vi "Main.vi"(11 "Module Admin":refnum<class "Delacor_lib_QMH_Cloneable Module Admin.lvclass">) -> ()   [LabVIEW 2020, in "FGen.lvlib"]
doc: "This template is based off of the Queued Message Handler design pattern and the Queued Message Handler project template that ships with LabVIEW.\n\nThe main difference is that the queue is private to this module and communication between modules is performed via Broadcast and Request events.\n\nRequest events are wrapped in public API methods and are handled in the Event Handling Loop (EHL) of this VI. Any module can register for Broadcast events sent by this module. The EHL generates messages based on user interface actions.\n\nThe Message Handling Loop (MHL) processes messages generated by the EHL, or by other messages. The messages are string values, so new messages can be added easily to the Message Cases case structure in the MHL. Each message cluster can also provide an optional value for Message Data, which is a variant that can be converted to whatever message-specific data is required.\n_____\nBased on DQMH Project Template 6.0.0.91."
uses:
  FGen.lvlib
  <vilib>/Delacor/Delacor QMH/Libraries/Message Queue_class/Delacor_lib_QMH_Message Queue.lvclass
  Module Data--cluster.ctl
  <vilib>/Utility/miscctls.llb/LVPointTypeDef.ctl
  <vilib>/Utility/error.llb/Error Cluster From Error Code.vi
  <vilib>/ErrorRing/Error Ring.xnode
  <vilib>/Delacor/Delacor QMH/Libraries/Message Queue_class/Delacor_lib_QMH_Enqueue Message (Single).vi
  Stop Argument--cluster.ctl
  <vilib>/Delacor/Delacor QMH/Libraries/Cloneable Module Admin_class/Delacor_lib_QMH_Cloneable Module Admin.lvclass
  Set Signal Type Argument--cluster.ctl
  Generador/Generador.lvclass
  Set to Default Argument--cluster.ctl
  Generate Signal (Reply Payload)--cluster.ctl
  Generate Signal Argument--cluster.ctl
panel:
  out "error out":errorcluster
  out "Status":string
  in  "Simulate EHL Error":bool
  in  "Simulate MHL Error":bool
  # "Other QMH Modules communicate with this Module via its Public API (wrappers for its Request Events).\n\nThis Module communicates with other Modules via its Broadcast Events.\nAny module that wants to get these messages, just registers for this module's Broadcast events."
  # "This template is for the Delacor Modified Queued Message Handler design pattern.\n\nSee the block diagram for more information on how to use this template."
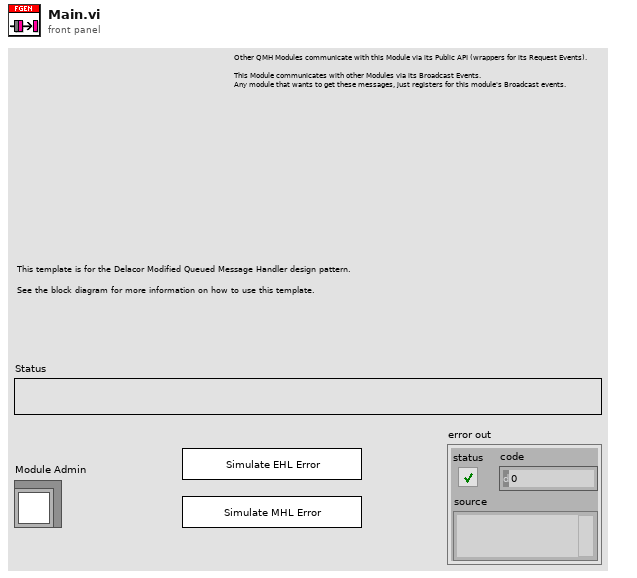
[diagram p1: front panel]
types:
  T1 = typedef "FGen.lvlib/Request Events--cluster.ctl" = cluster{"Stop Module":refnum<user-event>, "Show Panel":refnum<user-event>, "Hide Panel":refnum<user-event>, "Show Diagram":refnum<user-event>, "Get Module Execution Status":refnum<user-event>, "Set Signal Type":refnum<user-event>, "Set to Default":refnum<user-event>, "Generate Signal":refnum<user-event>}
  T2 = typedef "FGen.lvlib/Module Data--cluster.ctl" = cluster{"Status":string, "Generator":refnum<class "Generador.lvclass">}
  T3 = enum32{"invalid lock state", "Not Locked", "Locked (No Password)", "Password-protected"}
  T4 = typedef "FGen.lvlib/Stop Argument--cluster.ctl" = cluster{"Module ID":i32, "Origin":string, "Exit via Stop Module Req?":bool, "Wait for Module to stop?":bool}
  T5 = typedef "FGen.lvlib/Set Signal Type Argument--cluster.ctl" = cluster{"Module ID":i32, "signal type":enum16{"Sine Wave", "Triangle Wave", "Square Wave", "Sawtooth Wave"}}
  T6 = typedef "FGen.lvlib/Set to Default Argument--cluster.ctl" = cluster{"Module ID":i32, "Boolean":bool}
  T7 = typedef "FGen.lvlib/Generate Signal Argument--cluster.ctl" = cluster{"Module ID":i32, "Wait Notifier":refnum<notifier>, "wait for reply":bool}
  T8 = typedef "LVPointTypeDef.ctl" = cluster{"Horizontal":i16, "Vertical":i16}
  T9 = enum32{"Invalid", "Standard", "Closed", "Hidden", "Minimized", "Maximized"}
  T10 = typedef "FGen.lvlib/Generate Signal (Reply Payload)--cluster.ctl" = cluster{"signal out":waveform(dbl), "Generate Signal_error":errorcluster}
  T11 = enum16{"Sine Wave", "Triangle Wave", "Square Wave", "Sawtooth Wave"}
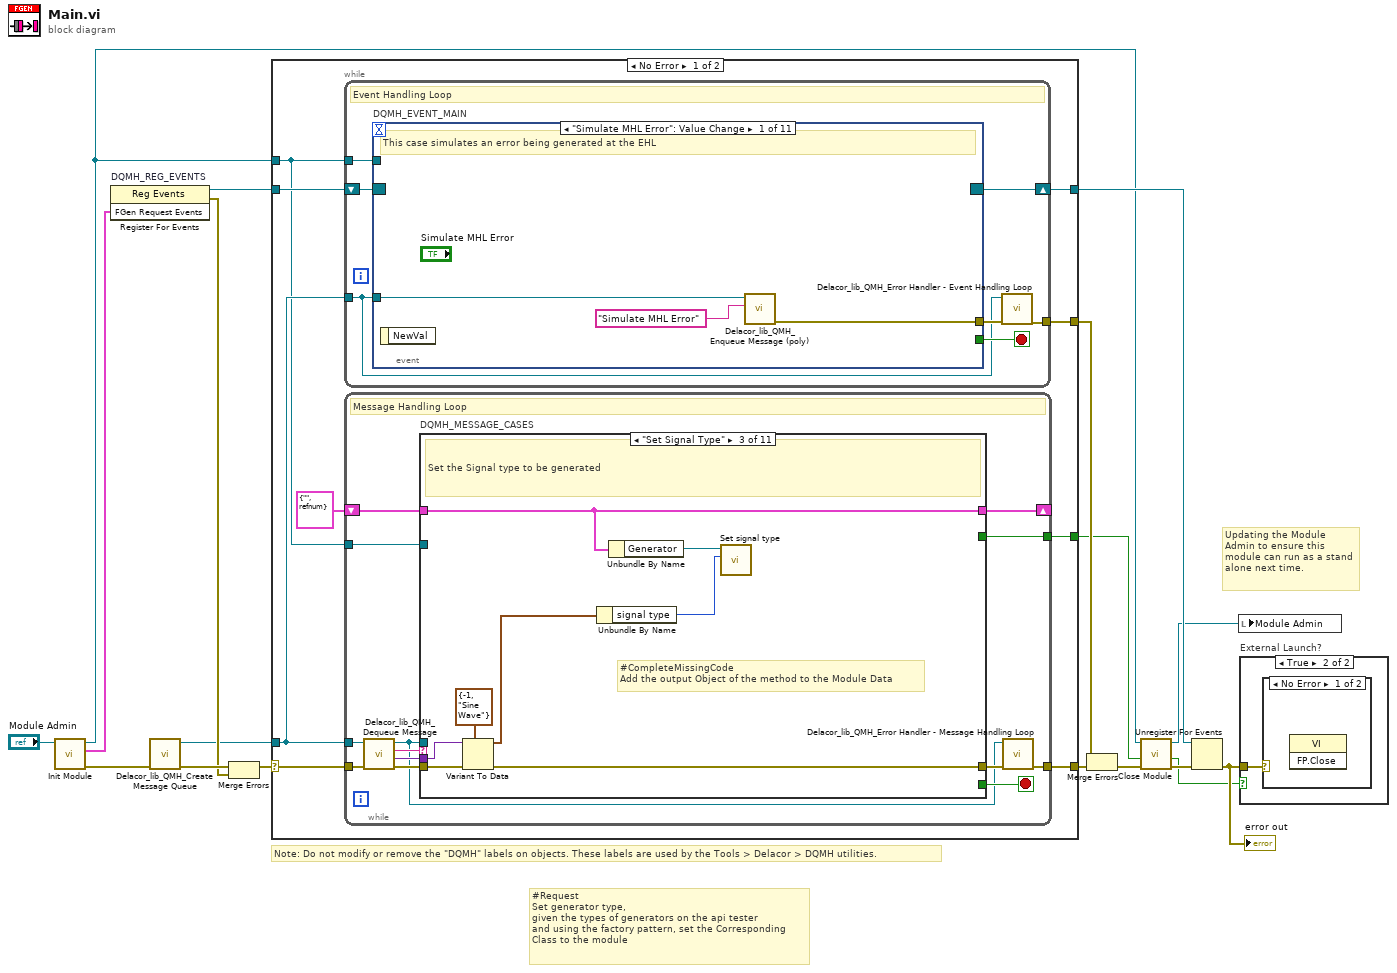
[diagram p0: block diagram]
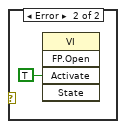
[diagram p3: hidden frame]
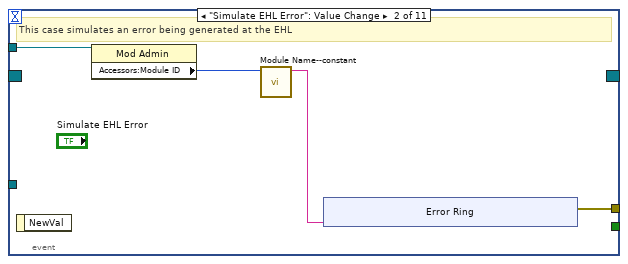
[diagram p4: hidden frame]
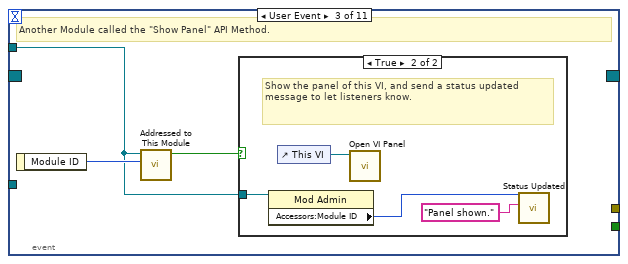
[diagram p5: hidden frame]
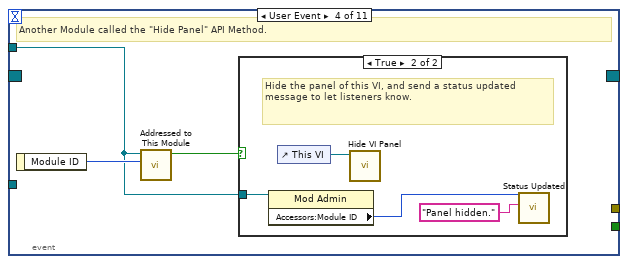
[diagram p7: hidden frame]
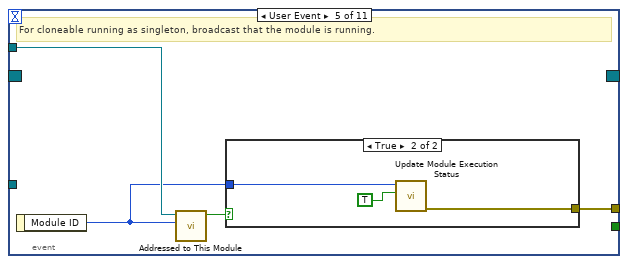
[diagram p9: hidden frame]
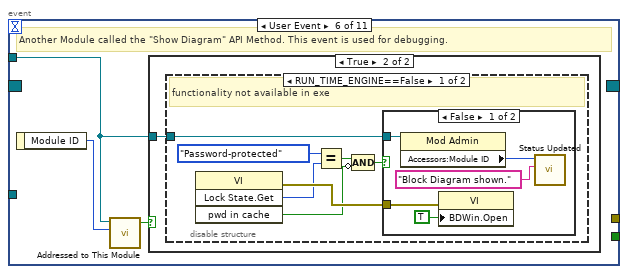
[diagram p11: hidden frame]
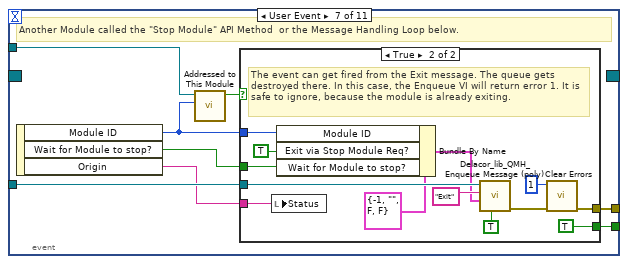
[diagram p15: hidden frame]
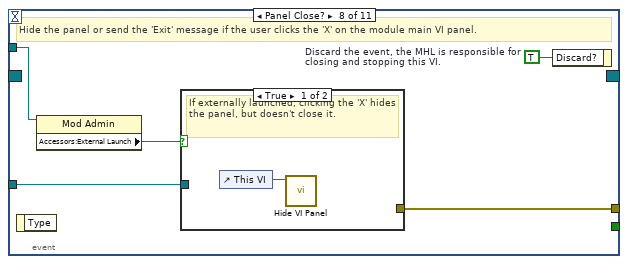
[diagram p17: hidden frame]
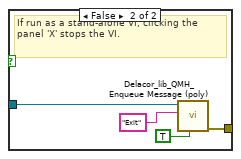
[diagram p18: hidden frame]
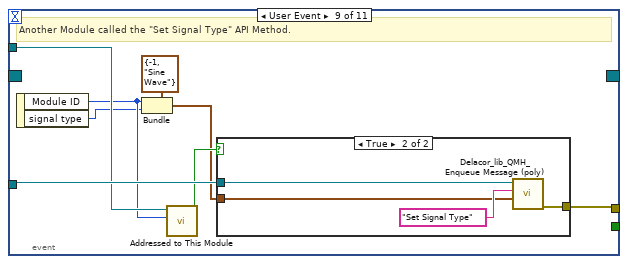
[diagram p19: hidden frame]
diagram:
  # "#Request\nSet generator type, \ngiven the types of generators on the api tester\nand using the factory pattern, set the Corresponding\nClass to the module"
  # "Note: Do not modify or remove the \"DQMH\" labels on objects. These labels are used by the Tools > Delacor > DQMH utilities."
  # "Updating the Module Admin to ensure this module can run as a stand alone next time."
  n1 = call "Init Module.vi"("Cloneable Module Admin in"="Module Admin") -> ("error out"=w15:errorcluster, "FGen Request Events"=w7:T1, "Cloneable Module Admin out"=w4:refnum<class "Delacor_lib_QMH_Cloneable Module Admin.lvclass">)  [unwired: 8 in]
  n2 = register-events "DQMH_REG_EVENTS"(w7) -> (reference out=w8:refnum<event-registration>, error out=w10:errorcluster)  [unwired: 2 in]
  n3 = call <vilib>:"Delacor_lib_QMH_Create Message Queue.vi"("error in"=w15) -> ("error out"=w12:errorcluster, "Message Queue"=w6:refnum<class "Delacor_lib_QMH_Message Queue.lvclass">)  [unwired: 9 in]
  n4 = Merge Errors(w12, w10) -> (w11:errorcluster)
  n5 = case shown="No Error" w11 {
    selector: w11 -> [w25 w290]
    tunnel: [w27 w289] -> w16
    tunnel: [w24 w297] -> w9
    tunnel: w8 -> [w22 w297]
    tunnel: w6 -> [w21 w288]
    tunnel: [w26 _] -> w17
    tunnel: w4 -> [w20 w293]
    tunnel: [w19 _] -> w2
    frame No Error {
      n6 = while {
        tunnel: w21 -> [w28]
        shift-right: [w31] -> w24
        shift-left: w22 -> [w32]
        tunnel: [w33] -> w26
        tunnel: w20 -> [w29]
        stop <- w30 stop-if-true
        # "Event Handling Loop"
        n7 = event "DQMH_EVENT_MAIN" shown="[0] \"Simulate MHL Error\": Value Change" {
          selector: w32 -> [_ _ _ _ _ _ _ _ _ _ _]
          dyn-events: [_ _ _ _ _ _ _ _ _ _ _] -> w31
          timeout: _ -> [_ _ _ _ _ _ _ _ _ _ _]
          tunnel: [_ _ _ _ _ _ w89 _ _ _ _] -> w30
          tunnel: w28 -> [w36 _ _ _ _ _ w92 w108 w124 w136 w149]
          tunnel: [w37 w41 _ _ w66 _ w93 w111 w117 w129 w141] -> w34
          tunnel: w29 -> [_ w40 w49 w56 w64 w70 w91 w109 w122 w134 w147]
          event "Simulate MHL Error": Value Change {
            # "This case simulates an error being generated at the EHL"
            n8 = event-data() -> ()  [unwired: 1 in, 1 out]
            n9 = call-poly <vilib>:"Delacor_lib_QMH_Enqueue Message (poly).vi"("Message"="Simulate MHL Error", "Message Queue in"=w36) -> ("error out"=w37:errorcluster)  [unwired: 8 in, 1 out]
          }
          event "Simulate EHL Error": Value Change {
            # "This case simulates an error being generated at the EHL"
            n10 = event-data() -> ()  [unwired: 1 in, 1 out]
            n11 = property class="Mod Admin"(reference=w40) -> ("Accessors:Module ID"=w39:i32)  [unwired: 1 in, 2 out]
            n12 = call "Module Name--constant.vi"("Module ID"=w39) -> ("Module Name"=w38:string)  [unwired: 10 in]
            n13 = xnode "Error Ring"("parameter 0"=w38) -> ("error out"=w41:errorcluster)
          }
          event User Event {
            # "Another Module called the \"Show Panel\" API Method."
            n14 = event-data() -> ("Module ID"=w50:i32)  [unwired: 1 in]
            n15 = call "Addressed to This Module.vi"("Module ID from Argument"=w50, "Module Admin"=w49) -> ("Addressed to this instance?"=w51:bool)  [unwired: 8 in, 1 out]
            n16 = case shown="True" w51 {
              tunnel: w49 -> [_ w53]
              frame False {
              }
              frame True {
                # "Show the panel of this VI, and send a status updated message to let listeners know."
                n17 = property class="Mod Admin"(reference=w53) -> ("Accessors:Module ID"=w52:i32)  [unwired: 1 in, 2 out]
                n18 = control-ref of="This VI"() -> (w55:refnum<vi>)
                n19 = call "Open VI Panel.vi"("VI"=w55) -> ()  [unwired: 10 in, 1 out]
                n20 = call "Status Updated.vi"("Status"="Panel shown." ("format string"), "Module ID"=w52) -> ()  [unwired: 9 in, 1 out]
              }
            }
          }
          event User Event {
            # "Another Module called the \"Hide Panel\" API Method."
            n21 = event-data() -> ("Module ID"=w57:i32)  [unwired: 1 in]
            n22 = call "Addressed to This Module.vi"("Module ID from Argument"=w57, "Module Admin"=w56) -> ("Addressed to this instance?"=w58:bool)  [unwired: 8 in, 1 out]
            n23 = case shown="True" w58 {
              tunnel: w56 -> [_ w60]
              frame False {
              }
              frame True {
                # "Hide the panel of this VI, and send a status updated message to let listeners know."
                n24 = property class="Mod Admin"(reference=w60) -> ("Accessors:Module ID"=w59:i32)  [unwired: 1 in, 2 out]
                n25 = control-ref of="This VI"() -> (w62:refnum<vi>)
                n26 = call "Hide VI Panel.vi"("VI"=w62) -> ()  [unwired: 10 in, 1 out]
                n27 = call "Status Updated.vi"("Status"="Panel hidden." ("format string"), "Module ID"=w59) -> ()  [unwired: 9 in, 1 out]
              }
            }
          }
          event User Event {
            # "For cloneable running as singleton, broadcast that the module is running."
            n28 = event-data() -> ("Module ID"=w63:i32)  [unwired: 1 in]
            n29 = call "Addressed to This Module.vi"("Module ID from Argument"=w63, "Module Admin"=w64) -> ("Addressed to this instance?"=w65:bool)  [unwired: 8 in, 1 out]
            n30 = case shown="True" w65 {
              tunnel: [_ w69] -> w66
              tunnel: w63 -> [_ w68]
              frame False {
              }
              frame True {
                n31 = call "Update Module Execution Status.vi"("Running?"=TRUE, "Module ID"=w68) -> ("error out"=w69:errorcluster)  [unwired: 9 in]
              }
            }
          }
          event User Event {
            # "Another Module called the \"Show Diagram\" API Method. This event is used for debugging."
            n32 = event-data() -> ("Module ID"=w71:i32)  [unwired: 1 in]
            n33 = call "Addressed to This Module.vi"("Module ID from Argument"=w71, "Module Admin"=w70) -> ("Addressed to this instance?"=w72:bool)  [unwired: 8 in, 1 out]
            n34 = case shown="True" w72 {
              tunnel: w70 -> [_ w73]
              frame False {
              }
              frame True {
                n35 = disable-structure shown="RUN_TIME_ENGINE==False" {
                  disable-tunnel: w73 -> [w74 _]
                  frame condition #0 (active) {
                    # "functionality not available in exe"
                    n36 = invoke class="VI" method="Lock State.Get"() -> (error out=w80:errorcluster, "Get Lock State"=w79:T3, "pwd in cache"=w76:bool)  [unwired: 4 in, 1 out]
                    n37 = Equal?(x=T3."Password-protected", y=w79) -> (x = y?=w77:bool)
                    n38 = Compound Arithmetic op=AND(w77, invert w76) -> (w75:bool)
                    n39 = case shown="False" w75 {
                      tunnel: w80 -> [w85 _]
                      tunnel: w74 -> [w82 _]
                      frame False {
                        n40 = property class="Mod Admin"(reference=w82) -> ("Accessors:Module ID"=w81:i32)  [unwired: 1 in, 2 out]
                        n41 = property class="VI"(error in=w85, "BDWin.Open"=TRUE ("Block Diagram Window:Open")) -> ()  [unwired: 1 in, 2 out]
                        n42 = call "Status Updated.vi"("Status"="Block Diagram shown." ("format string"), "Module ID"=w81) -> ()  [unwired: 9 in, 1 out]
                      }
                      frame True {
                        # "Password-protected VI, and the password is not in the cache. Do not show the diagram."
                      }
                    }
                  }
                  frame condition #1 {
                  }
                }
              }
            }
          }
          event User Event {
            # "Another Module called the \"Stop Module\" API Method  or the Message Handling Loop below."
            n43 = event-data() -> ("Module ID"=w87:i32, "Wait for Module to stop?"=w88:bool, "Origin"=w86:string)  [unwired: 1 in]
            n44 = call "Addressed to This Module.vi"("Module ID from Argument"=w87, "Module Admin"=w91) -> ("Addressed to this instance?"=w90:bool)  [unwired: 8 in, 1 out]
            n45 = case shown="True" w90 {
              tunnel: [_ w105] -> w93
              tunnel: w92 -> [_ w101]
              tunnel: [_ TRUE] -> w89
              tunnel: w88 -> [_ w96]
              tunnel: w87 -> [_ w98]
              tunnel: w86 -> [_ w94]
              frame False {
              }
              frame True {
                # "The event can get fired from the Exit message. The queue gets destroyed there. In this case, the Enqueue VI will return error 1. It is safe to ignore, because the module is already exiting."
                n46 = local write "Status"(w94) -> ()
                n47 = Bundle By Name(cluster=T4 {"Module ID"=-1, "Origin"="", "Exit via Stop Module Req?"=FALSE, "Wait for Module to stop?"=FALSE} ("Stop Argument"), "Module ID"=w98, "Exit via Stop Module Req?"=TRUE, "Wait for Module to stop?"=w96) -> (w95:T4)
                n48 = call-poly <vilib>:"Delacor_lib_QMH_Enqueue Message (poly).vi"("Priority Message? (F)"=TRUE, "Message Data"=w95, "Message"="Exit", "Message Queue in"=w101) -> ("error out"=w106:errorcluster)  [unwired: 6 in, 1 out]
                n49 = call <vilib>:"Clear Errors.vi"("error in (no error)"=w106, "specific error code to clear (0: all)"=1) -> ("error out"=w105:errorcluster)  [unwired: 4 in, 1 out]
              }
            }
          }
          event Panel Close? {
            w110 = TRUE  # Discard the event, the MHL is responsible for closing and stopping this VI.
            # "Hide the panel or send the 'Exit' message if the user clicks the 'X' on the module main VI panel."
            n50 = event-data() -> ()  [unwired: 1 in, 1 out]
            n51 = property class="Mod Admin"(reference=w109) -> ("Accessors:External Launch"=w107:bool)  [unwired: 1 in, 2 out]
            n52 = case shown="True" w107 {
              tunnel: w108 -> [_ w115]
              tunnel: [_ w116] -> w111
              frame True {
                # "If externally launched, clicking the 'X' hides the panel, but doesn't close it."
                n53 = control-ref of="This VI"() -> (w112:refnum<vi>)
                n54 = call "Hide VI Panel.vi"("VI"=w112) -> ()  [unwired: 10 in, 1 out]
              }
              frame False {
                # "If run as a stand-alone VI, clicking the panel 'X' stops the VI."
                n55 = call-poly <vilib>:"Delacor_lib_QMH_Enqueue Message (poly).vi"("Priority Message? (F)"=TRUE, "Message"="Exit", "Message Queue in"=w115) -> ("error out"=w116:errorcluster)  [unwired: 7 in, 1 out]
              }
            }
            n56 = event-data("Discard?"=w110) -> ()  [unwired: 1 in, 1 out]
          }
          event User Event {
            # "Another Module called the \"Set Signal Type\" API Method."
            n57 = event-data() -> ("Module ID"=w119:i32, "signal type"=w118:T11)  [unwired: 1 in]
            n58 = Bundle(cluster=T5 {"Module ID"=-1, "signal type"=enum."Sine Wave"} ("Set Signal Type Argument"), "Module ID"=w119, "signal type"=w118) -> (w120:T5)
            n59 = call "Addressed to This Module.vi"("Module ID from Argument"=w119, "Module Admin"=w122) -> ("Addressed to this instance?"=w123:bool)  [unwired: 8 in, 1 out]
            n60 = case shown="True" w123 {
              tunnel: w124 -> [_ w128]
              tunnel: w120 -> [_ w126]
              tunnel: [_ w125] -> w117
              frame False {
              }
              frame True {
                n61 = call-poly <vilib>:"Delacor_lib_QMH_Enqueue Message (poly).vi"("Message Data"=w126, "Message"="Set Signal Type", "Message Queue in"=w128) -> ("error out"=w125:errorcluster)  [unwired: 7 in, 1 out]
              }
            }
          }
          event User Event {
            # "Another Module called the \"Set to Default\" API Method."
            n62 = event-data() -> ("Module ID"=w131:i32, "Boolean"=w130:bool)  [unwired: 1 in]
            n63 = Bundle(cluster=T6 {"Module ID"=-1, "Boolean"=FALSE} ("Set to Default Argument"), "Module ID"=w131, "Boolean"=w130) -> (w132:T6)
            n64 = call "Addressed to This Module.vi"("Module ID from Argument"=w131, "Module Admin"=w134) -> ("Addressed to this instance?"=w135:bool)  [unwired: 8 in, 1 out]
            n65 = case shown="True" w135 {
              tunnel: w136 -> [_ w140]
              tunnel: w132 -> [_ w138]
              tunnel: [_ w137] -> w129
              frame False {
              }
              frame True {
                n66 = call-poly <vilib>:"Delacor_lib_QMH_Enqueue Message (poly).vi"("Message Data"=w138, "Message"="Set to Default", "Message Queue in"=w140) -> ("error out"=w137:errorcluster)  [unwired: 7 in, 1 out]
              }
            }
          }
          event User Event {
            # "Another Module called the \"Generate Signal\" API Method."
            n67 = event-data() -> ("Module ID"=w144:i32, "Wait Notifier"=w143:refnum<notifier>, "wait for reply"=w142:bool)  [unwired: 1 in]
            n68 = Bundle(cluster=T7 {"Module ID"=-1, "Wait Notifier"=refnum, "wait for reply"=FALSE} ("Generate Signal Argument"), "Module ID"=w144, "Wait Notifier"=w143, "wait for reply"=w142) -> (w145:T7)
            n69 = call "Addressed to This Module.vi"("Module ID from Argument"=w144, "Module Admin"=w147) -> ("Addressed to this instance?"=w148:bool)  [unwired: 8 in, 1 out]
            n70 = case shown="True" w148 {
              tunnel: w149 -> [_ w153]
              tunnel: w145 -> [_ w151]
              tunnel: [_ w150] -> w141
              frame False {
              }
              frame True {
                n71 = call-poly <vilib>:"Delacor_lib_QMH_Enqueue Message (poly).vi"("Message Data"=w151, "Message"="Generate Signal", "Message Queue in"=w153) -> ("error out"=w150:errorcluster)  [unwired: 7 in, 1 out]
              }
            }
          }
        }
        n72 = call-dynamic "Delacor_lib_QMH_Error Handler - Event Handling Loop.vi"("error in"=w34, "Message Queue in"=w28) -> ("dup error in"=w33:errorcluster)  [unwired: 8 in, 1 out]
      }
      n73 = while {
        tunnel: w21 -> [w157]
        shift-right: [w161] -> _
        shift-left: T2 {"Status"="", "Generator"=refnum} ("Data Cluster") -> [w162]
        tunnel: w25 -> [w165]
        tunnel: [w163] -> w27
        tunnel: w20 -> [w155]
        tunnel: [w154] -> w19
        stop <- w160 stop-if-true
        # "Message Handling Loop"
        n74 = call-dynamic "Delacor_lib_QMH_Dequeue Message.vi"("error in"=w165, "Message Queue in"=w157) -> ("error out"=w164:errorcluster, "Message Data"=w158:variant, "Message"=w159:string, "Message Queue out"=w156:refnum<class "Delacor_lib_QMH_Message Queue.lvclass">)  [unwired: 6 in]
        n75 = case "DQMH_MESSAGE_CASES" shown="\"Set Signal Type\"" w159 {
          selector: w159 -> [_ _ _ _ _ _ _ _ _ _ w275]
          tunnel: w156 -> [_ _ _ _ _ _ _ w226 _ w265 _]
          tunnel: w164 -> [w185 w189 w197 w204 w217 w222 w224 w235 w248 w271 w277]
          tunnel: [w183 w189 w196 w203 w207 w221 w224 w231 w247 w268 w278] -> w166
          tunnel: w162 -> [w176 w188 w192 w199 w216 w220 w223 w230 w245 w264 w276]
          tunnel: [w175 w188 w192 w199 w216 w220 w223 w230 w245 w264 w276] -> w161
          tunnel: [_ _ _ _ _ _ _ _ _ w263 _] -> w160
          tunnel: w158 -> [_ _ w195 w202 w214 _ _ w229 _ w261 _]
          tunnel: w155 -> [w170 _ _ _ _ _ _ w228 w243 w257 w273]
          tunnel: [_ _ _ _ _ _ _ _ _ w259 _] -> w154
          frame "Initialize" {
            w167 = "Initial Message" ("Initial Message")
            # "#Factory_Pattern\nCreate a factory pattern and a broadcast\nto populate the clases Generador"
            # "Initialize - Any operation that needs to be done before the module can receive messages. Synchronize Caller Events.vi will inform Start Module.vi that the module has launched and is ready to receive messages. Module Did Init.vi will broadcast that the module initialized."
            n76 = call "Synchronize Caller Events.vi"("error in (no error)"=w185, "Module Admin"=w170) -> ("error out"=w184:errorcluster, "Module Admin out"=w169:refnum<class "Delacor_lib_QMH_Cloneable Module Admin.lvclass">)  [unwired: 8 in]
            n77 = property class="Mod Admin"(reference=w169) -> ("Accessors:Module ID"=w172:i32, "Accessors:External Launch"=w171:bool)  [unwired: 1 in, 2 out]
            n78 = call "Module Name--constant.vi"("Module ID"=w172) -> ("Module Name"=w180:string)  [unwired: 10 in]
            n79 = property class="VI"("Front Panel.Title"=w180) -> (reference out=w182:refnum<vi>, error out=w187:errorcluster)  [unwired: 2 in]
            n80 = Select(t=T9."Hidden" ("State"), s=w171, f=T9."Standard" ("State")) -> (s? t:f=w177:T9)
            n81 = invoke class="VI" method="FP.Open"(reference=w182, error in=w187, "State"=w177) -> (reference out=w181:refnum<vi>, error out=w186:errorcluster)  [unwired: 2 in, 3 out]
            n82 = call "Module Name--constant.vi"("Module ID"=w172) -> ("Module Name"=w173:string)  [unwired: 10 in]
            n83 = Bundle By Name(cluster=w176, "Status"=w167) -> (w175:T2)
            n84 = invoke class="VI" method="FP.Center"(reference=w181, error in=w186) -> ()  [unwired: 1 in, 3 out]
            n85 = property on="Pane" class="Pane"("Origin"=T8 {"Horizontal"=0, "Vertical"=0}) -> ()  [unwired: 2 in, 2 out]
            n86 = call "Module Did Init.vi"("error in (no error)"=w184, "Initialized?"=TRUE, "Origin"=w173, "Module ID"=w172) -> ("error out"=w183:errorcluster)  [unwired: 7 in]
            "Status" <- w167
          }
          frame "---Module Specific---" {
            # "Separator -- The following cases handle messages specific to this Module."
          }
          frame "Set Signal Type" {
            # "#CompleteMissingCode\nAdd the output Object of the method to the Module Data"
            # "Set the Signal type to be generated"
            n87 = Variant To Data(error in=w197, type=T5 {"Module ID"=-1, "signal type"=enum."Sine Wave"} ("Set Signal Type Argument"), Variant=w195) -> (data=w193:T5, error out=w196:errorcluster)
            n88 = Unbundle By Name(w193) -> ("signal type"=w190:T11)
            n89 = Unbundle By Name(w192) -> ("Generator"=w191:refnum<class "Generador.lvclass">)
            n90 = call "Set signal type.vi"("signal type"=w190, "Generator in"=w191) -> ()  [unwired: 8 in, 2 out]
          }
          frame "Set to Default" {
            # "#CompleteMissingCode\nAdd the output Object of the method to the Module Data"
            # "Set the signal to default values"
            n91 = Variant To Data(error in=w204, type=T6 {"Module ID"=-1, "Boolean"=FALSE} ("Set to Default Argument"), Variant=w202) -> (data=w200:T6, error out=w203:errorcluster)
            n92 = Unbundle By Name(w200) -> ()  [unwired: 2 out]
            n93 = Unbundle By Name(w199) -> ("Generator"=w198:refnum<class "Generador.lvclass">)
            n94 = call-dynamic "Default--constant.vi"("Generator in"=w198) -> ()  [unwired: 9 in, 2 out]
          }
          frame "Generate Signal" {
            # "#CompleteMissingCode\nAdd the class to the method"
            # "Generate the signal with the Defined values"
            n95 = Variant To Data(error in=w217, type=T7 {"Module ID"=-1, "Wait Notifier"=refnum, "wait for reply"=FALSE} ("Generate Signal Argument"), Variant=w214) -> (data=w212:T7, error out=w215:errorcluster)
            n96 = Unbundle By Name(w212) -> ("Wait Notifier"=w211:refnum<notifier>, "wait for reply"=w210:bool)  [unwired: 1 out]
            n97 = call "Generate Waveform.vi"("Generator in"=refnum<class "Generador.lvclass"> refnum ("FGen.lvlib:Generator")) -> ("Waveform"=w206:waveform(dbl))  [unwired: 8 in, 2 out]
            n98 = Bundle By Name(cluster=T10 {"signal out"={"t0"=timestamp(0 s since 1904-01-01), "dt"=1.0, "Y"=[]}, "Generate Signal_error"={"status"=FALSE, "code"=0, "source"=""}} ("Generate Signal (Reply Payload)"), "signal out"=w206) -> (w209:T10)  [unwired: 1 in]
            n99 = case shown="True" w210 {
              tunnel: w211 -> [_ w219]
              tunnel: w209 -> [_ w218]
              frame False {
              }
              frame True {
                n100 = Send Notification(notification=w218, notifier=w219) -> ()  [unwired: 1 in, 2 out]
              }
            }
            n101 = Merge Errors(w215) -> (w207:errorcluster)  [unwired: 1 in]
          }
          frame "---Copy This Frame---" {
            # "Duplicate this frame when creating new messages.  Change this comment in the duplicated frame to describe this message."
            n102 = Merge Errors(w222) -> (w221:errorcluster)
          }
          frame "---Exit and Error Handling---" {
            # "Separator - the following cases handle errors and exit messages."
          }
          frame "Error" {
            # "Error - Check the error message data and respond accordingly. This message is sent by the \"Error Handler\" VIs at the end of each loop in this application."
            n103 = property class="Mod Admin"(reference=w228) -> ("Accessors:External Launch"=w227:bool, "Accessors:Module ID"=w225:i32)  [unwired: 1 in, 2 out]
            n104 = Variant To Data(error in=w235, type=errorcluster {"status"=FALSE, "code"=0, "source"=""} ("error constant"), Variant=w229) -> (data=w236:errorcluster, error out=w233:errorcluster)
            n105 = call "Error Reported.vi"("Error"=w236, "Module ID"=w225) -> ()  [unwired: 9 in, 1 out]
            n106 = case shown="False" w227 {
              tunnel: [w241 _] -> w232
              tunnel: w226 -> [w239 _]
              tunnel: w236 -> [w240 _]
              frame False {
                # "If the module is running standalone, then pop up an error dialog and call the \"Exit\" message."
                n107 = call <vilib>:"Simple Error Handler.vi"("error in (no error)"=w240) -> ()  [unwired: 4 in, 5 out]
                n108 = call-poly <vilib>:"Delacor_lib_QMH_Enqueue Message (poly).vi"("Priority Message? (F)"=TRUE, "Message"="Exit", "Message Queue in"=w239) -> ("error out"=w241:errorcluster)  [unwired: 7 in, 1 out]
              }
              frame True {
                # "If the module was launched externally, calling the Error Reported broadcast VI is the only action performed by the \"Error\" message. The module's caller can then process the error appropriately."
              }
            }
            n109 = Merge Errors(w233, w232) -> (w231:errorcluster)
            n110 = local write "error out"(w231) -> ()
          }
          frame "Simulate MHL Error" {
            # "Simulate an error occurring at the MHL"
            n111 = property class="Mod Admin"(reference=w243) -> ("Accessors:Module ID"=w244:i32)  [unwired: 1 in, 2 out]
            n112 = call "Module Name--constant.vi"("Module ID"=w244) -> ("Module Name"=w242:string)  [unwired: 10 in]
            n113 = xnode "Error Ring"("parameter 0"=w242) -> ("error out"=w246:errorcluster)
            n114 = Merge Errors(w248, w246) -> (w247:errorcluster)
          }
          frame "Exit" {
            w262 = 91  # 91: not all Exit messages will have an argument
            w263 = TRUE  # Stop the VI
            # "Release the message queue reference"
            # "Exit - Exit the application."
            n115 = Variant To Data(error in=w271, type=T4 {"Module ID"=-1, "Origin"="", "Exit via Stop Module Req?"=FALSE, "Wait for Module to stop?"=FALSE} ("Stop Argument"), Variant=w261) -> (data=w258:T4, error out=w266:errorcluster)
            n116 = call <vilib>:"Clear Errors.vi"("error in (no error)"=w266, "specific error code to clear (0: all)"=w262) -> ("error out"=w270:errorcluster)  [unwired: 4 in, 1 out]
            n117 = control-ref of="This VI"() -> (w256:refnum<vi>)
            n118 = call-dynamic "Delacor_lib_QMH_Release Message Queue.vi"("error in"=w270, "Message Queue"=w265) -> ("error out"=w269:errorcluster)  [unwired: 9 in]
            n119 = call "Handle Exit.vi"("Stop Argument"=w258, "Module Admin in"=w257, "VI reference"=w256) -> ("error out"=w267:errorcluster, "Wait for Stop?"=w259:bool)  [unwired: 7 in]
            n120 = Merge Errors(w269, w267) -> (w268:errorcluster)
          }
          frame Default {
            # "'Default' case only runs if there is a message that isn't defined in any of the other cases.  Output a programming error."
            n121 = property class="Mod Admin"(reference=w273) -> ("Accessors:Module ID"=w272:i32)  [unwired: 1 in, 2 out]
            n122 = call "Module Name--constant.vi"("Module ID"=w272) -> ("Module Name"=w274:string)  [unwired: 10 in]
            n123 = xnode "Error Ring"("parameter 0"=w275, "parameter 1"=w274) -> ("error out"=w279:errorcluster)
            n124 = Merge Errors(w277, w279) -> (w278:errorcluster)
          }
        }
        n125 = call-dynamic "Delacor_lib_QMH_Error Handler - Message Handling Loop.vi"("error in"=w166, "Message Queue in"=w156) -> ("dup error in"=w163:errorcluster)  [unwired: 8 in, 1 out]
      }
    }
    frame Error {
      n126 = call "Synchronize Caller Events.vi"("Module Admin"=w293) -> ("Module Admin out"=w292:refnum<class "Delacor_lib_QMH_Cloneable Module Admin.lvclass">)  [unwired: 9 in, 1 out]
      n127 = property class="Mod Admin"(reference=w292) -> ("Accessors:Module ID"=w291:i32)  [unwired: 1 in, 2 out]
      n128 = call-dynamic "Delacor_lib_QMH_Release Message Queue.vi"("error in"=w290, "Message Queue"=w288) -> ("error out"=w289:errorcluster)  [unwired: 9 in]
      n129 = call "Module Name--constant.vi"("Module ID"=w291) -> ("Module Name"=w296:string)  [unwired: 10 in]
      n130 = Format Into String(format string="An error occurred during initialization. %s is no longer running.", w296) -> (resulting string=w294:string)  [unwired: 2 in, 1 out]
      n131 = call "Error Reported.vi"("Additional Information"=w294, "Error"=w289, "Module ID"=w291) -> ()  [unwired: 8 in, 1 out]
    }
  }
  n132 = Merge Errors(w17, w16) -> (w18:errorcluster)
  n133 = call "Close Module.vi"("error in"=w18, "Wait for stop?"=w2, "Module Admin in"=w4) -> ("error out"=w14:errorcluster, "External Launch"=w1:bool, "Module Admin out"=w3:refnum<class "Delacor_lib_QMH_Cloneable Module Admin.lvclass">)  [unwired: 6 in]
  n134 = Unregister For Events(event registration refnum=w9, error in=w14) -> (error out=w13:errorcluster)
  "error out" <- w13
  n135 = local write "Module Admin"(w3) -> ()
  n136 = case "External Launch?" shown="True" w1 {
    tunnel: w13 -> [_ w298]
    frame False {
    }
    frame True {
      n137 = case shown="No Error" w298 {
        frame No Error {
          n138 = invoke class="VI" method="FP.Close"() -> ()  [unwired: 3 in, 3 out]
        }
        frame Error {
          n139 = invoke class="VI" method="FP.Open"("Activate"=TRUE ("Activate?")) -> ()  [unwired: 4 in, 5 out]
        }
      }
    }
  }
